vi "OneTimeCalib.vi"(8 "error in":errorcluster, 11 "MagSpec_Bella in":refnum<class "MagSpec_Bella.lvclass">) -> (0 "error out":errorcluster, 3 "MagSpec_Bella out":refnum<class "MagSpec_Bella.lvclass">)   [LabVIEW 2020, in "MagSpec_Bella.lvclass"]
uses:
  MagSpec_Bella.lvclass
  OnOffTypeDef.ctl
  MagSpec_Bella.lvclass/MagSpec_Bella.ctl
  OneTimeCalculation.ctl
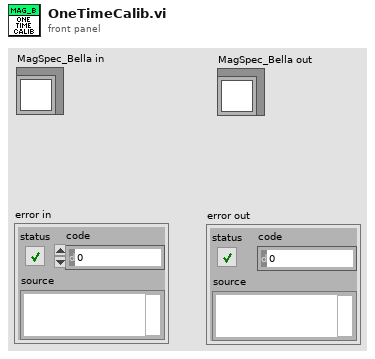
[diagram p1: front panel]
types:
  T1 = typedef "OnOffTypeDef.ctl" = enum16{"off", "on"}
  T2 = typedef "CameraSettings_File.ctl" = cluster{"FOV [mm]":dbl, "Left edge [mm]":dbl, "ROI Y offset":dbl, "ROI height":dbl, "ROI X offset":dbl, "ROI width":dbl, "Y center pixel":dbl, "Y Start":dbl, "Y End":dbl, "X Start":dbl, "X End":dbl, "rot [deg]":dbl}
  T3 = typedef "OneTimeCalculation.ctl" = cluster{"first Pixel pos [m]":dbl, "Pixel Size [mm]":dbl, "forward":T1}
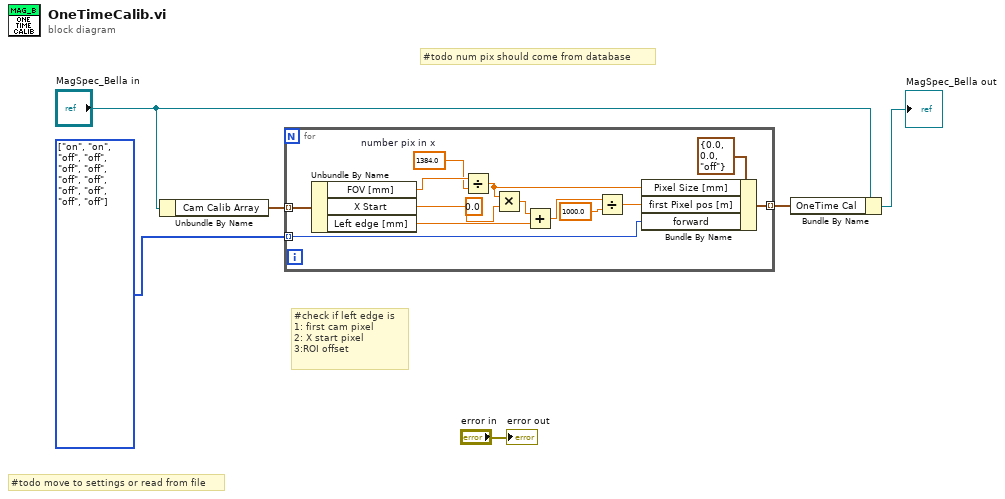
[diagram p0: block diagram]
diagram:
  w1 = T1[] [enum."on", enum."on", enum."off", enum."off", enum."off", enum."off", enum."off", enum."off", enum."off", enum."off", enum."off", enum."off"] items=["off", "on"]
  # "#todo num pix should come from database"
  # "#check if left edge is \n1: first cam pixel \n2: X start pixel\n3:ROI offset"
  # "#todo move to settings or read from file"
  n1 = Unbundle By Name("MagSpec_Bella in") -> ("Cam Calib Array"=w3:T2[])
  n2 = for {
    tunnel: w3 -> [w19] mode=indexing
    tunnel: [w15] -> w5 mode=indexing
    tunnel: w1 -> [w8] mode=indexing
    (unwired) 0.0 ("y")
    w16 = 1384.0  # number pix in x
    n3 = Unbundle By Name(w19) -> ("FOV [mm]"=w18:dbl, "X Start"=w7:dbl, "Left edge [mm]"=w11:dbl)
    n4 = Divide(x=w18, y=w16) -> (x/y=w10:dbl)
    n5 = Multiply(x=w10, y=w7) -> (x*y=w14:dbl)
    n6 = Add(x=w14, y=w11) -> (x+y=w13:dbl)
    n7 = Divide(x=w13, y=1000.0) -> (x/y=w9:dbl)
    n8 = Bundle By Name(cluster=T3 {"first Pixel pos [m]"=0.0, "Pixel Size [mm]"=0.0, "forward"=enum."off"} ("One time calculation"), "Pixel Size [mm]"=w10, "first Pixel pos [m]"=w9, "forward"=w8) -> (w15:T3)
  }
  n9 = Bundle By Name(cluster="MagSpec_Bella in", "OneTime Cal"=w5) -> (→"MagSpec_Bella out":refnum<class "MagSpec_Bella.lvclass">)
  "error out" <- "error in"
